vi "Write Measured Current.vi"(8 "error in (no error)":errorcluster, 10 "Raw_Current":u8, 11 "ProXR in":refnum<class "ProXR.lvclass">) -> (0 "error out":errorcluster, 3 "ProXR out":refnum<class "ProXR.lvclass">)   [LabVIEW 2019, in "ProXR.lvlib" / "ProXR.lvclass"]
uses:
  Library/ProXR.lvclass
  C:/Users/Public/Documents/Development/builds/Instruments/DIG_IO.lvlibp/Library/DIG_IO.lvclass
  builds/Instruments/DIG_IO.lvlibp/Accessors/Read Detected_Current_ref.vi
  builds/Instruments/DIG_IO.lvlibp/Accessors/Write Detected_Current_ref.vi
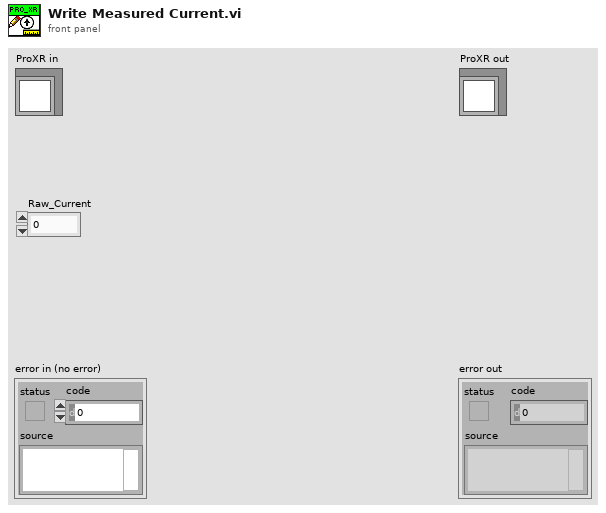
[diagram p1: front panel]
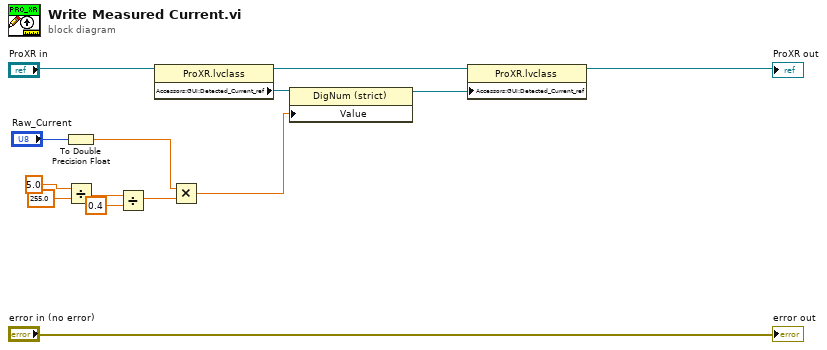
[diagram p0: block diagram]
diagram:
  n1 = To Double Precision Float(number="Raw_Current") -> (double precision float=w4:dbl)
  n2 = Divide(x=5.0, y=255.0) -> (x/y=w7:dbl)
  n3 = Divide(x=w7, y=0.4) -> (x/y=w5:dbl)
  n4 = property class="ProXR.lvclass"(reference="ProXR in") -> (reference out=w11:refnum<class "ProXR.lvclass">, "Accessors:GUI:Detected_Current_ref"=w10:refnum<vi>)  [unwired: 1 in, 1 out]
  n5 = Multiply(x=w4, y=w5) -> (x*y=w3:dbl)
  n6 = property class="DigNum (strict)"(reference=w10, "Value"=w3) -> (reference out=w1:refnum<vi>)  [unwired: 1 in, 1 out]
  n7 = property class="ProXR.lvclass"(reference=w11, "Accessors:GUI:Detected_Current_ref"=w1) -> (reference out=→"ProXR out":refnum<class "ProXR.lvclass">)  [unwired: 1 in, 1 out]
  "error out" <- "error in (no error)"
